vi "Close.vi"(8 "error in (no error)":errorcluster) -> (0 "error out":errorcluster)   [LabVIEW 2019, in "Kinova MICO² USB.lvlib"]
uses:
  <vilib>/Utility/error.llb/Error Cluster From Error Code.vi
  <vilib>/ErrorRing/Error Ring.xnode
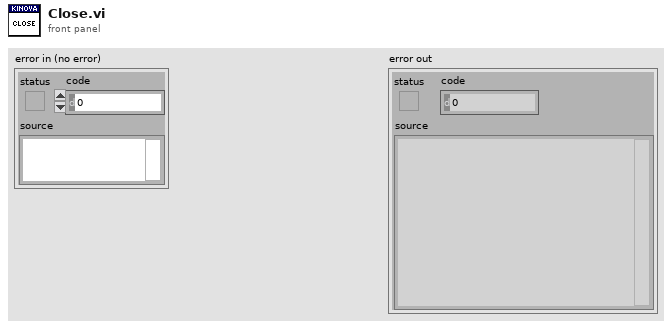
[diagram p1: front panel]
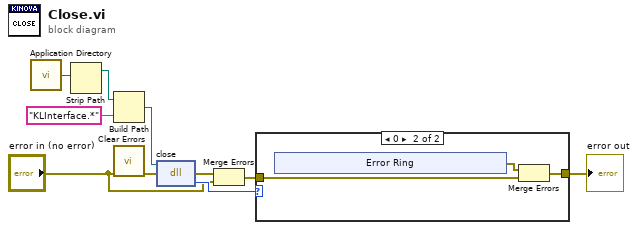
[diagram p0: block diagram]
diagram:
  n1 = call <vilib>:"Application Directory.vi"() -> ("Application Directory"=w1:path)
  n2 = Strip Path(path=w1) -> (stripped path=w8:path)  [unwired: 1 out]
  n3 = Build Path(base path=w8, name or relative path="KLInterface.*") -> (appended path=w2:path)
  n4 = call <vilib>:"Clear Errors.vi"("error in (no error)"="error in (no error)") -> ("error out"=w6:errorcluster)  [unwired: 5 in, 1 out]
  n5 = dll-call lib="C:/Users/mcjssdcc/source/repos/Kinova Labview Interface/Debug/KLInterface.dll" fn="close"(path in=w2, error in=w6) -> (error out=w4:errorcluster, "return type"=w9:i32)  [unwired: 1 in, 1 out]
  n6 = Merge Errors(w4, "error in (no error)") -> (w3:errorcluster)
  n7 = case shown="0" w9 {
    tunnel: [w11 w13] -> w7
    tunnel: w3 -> [w11 w12]
    frame 1, Default {
    }
    frame 0 {
      n8 = xnode "Error Ring"() -> ("error out"=w14:errorcluster)
      n9 = Merge Errors(w14, w12) -> (w13:errorcluster)
    }
  }
  "error out" <- w7
